vi "ATF-P&ID v2.vi"() -> ()   [LabVIEW 2022 SP3]
panel:
  in  "Exit":bool
  out "Boolean 73":bool
  out "Boolean 30":bool
  in  "F EPV 1008":bool
  out "NC EPV 1008 HSS":bool
  out "Boolean 27":bool
  in  "F EPV 1007":bool
  out "F EPV 1007 HSS":bool
  in  "F EPV 1004":bool
  out "NC EPV 1004 HSS":bool
  out "Boolean 26":bool
  in  "NC EPV 1001":bool
  out "NC EPV 1001 HSS":bool
  out "Boolean 23":bool
  out "Boolean 25":bool
  out "NO EPV 477 HSS  3":bool
  in  "NC EPV 61":bool
  out "Boolean 104":bool
  out "Boolean 47":bool
  out "Boolean 3":bool
  out "Boolean 24":bool
  out "NC EPV 56 HSS":bool
  in  "NC EPV 56":bool
  out "Boolean 16":bool
  out "Boolean 116":bool
  in  "NO EPV 122":bool
  out "Boolean 46":bool
  out "NO EPV 1102 HSS 2":bool
  out "Boolean 103":bool
  out "F_RTD_56(K)":dbl format="%.2g"
  out "N_PT_121":dbl format="%.2g"
  out "WTT_LS 2":dbl(slide) scale=0.1..100.0
  out "Boolean 71":bool
  out "F_RTD_1013 (K)":dbl format="%.2g"
  out "PT SC":dbl format="%.2g"
  out "W_RTD_1177 (K)":dbl format="%.2g"
  out "F_SC_RTD(K)":dbl format="%.2g"
  out "PT 1000(K)":dbl format="%.2g"
  out "PT 1000-2 (K)":dbl format="%.2g"
  out "F_PT_1013b (bar)":dbl format="%.2g"
  out "F_PT_1013a (bar)":dbl format="%.2g"
  out "F_PT_1019":dbl format="%.2g"
  out "F_TCV_1018":dbl format="%.2g"
  out "TCV_1018(FB) %":dbl format="%.2g"
  out "Boolean 108":bool
  out "Boolean 107":bool
  out "F_RTD_1011(K)":dbl format="%.2g"
  out "Boolean 21":bool
  out "Boolean 138":bool
  out "Boolean 29":bool
  out "Boolean 28":bool
  out "F_PT_1011a (bar)":dbl format="%.2g"
  out "F_PT_1011b (bar)":dbl format="%.2g"
  out "F_FM_1010 (kg/s)":dbl format="%.2g"
  out "Boolean 106":bool
  out "Boolean 105":bool
  out "Boolean 121":bool
  out "Boolean 126":bool
  out "Boolean 109":bool
  out "Boolean 6":bool
  out "Boolean 81":bool
  out "NO EPV 477 HSS  2":bool
  in  "NO EPV 477":bool
  in  "NO EPV 478R":bool
  out "NO EPV 1207 HSS 2":bool
  out "Boolean 54":bool
  out "Boolean 53":bool
  out "Boolean 22":bool
  out "Boolean 86":bool
  out "F_PT_56 _R":dbl format="%.2g"
  in  "NC EPV 481":bool
  out "NC EPV 481 HSS":bool
  out "Boolean 85":bool
  out "F_PT_56":dbl format="%.2g"
  out "Boolean 115":bool
  out "Boolean 52":bool
  out "N_PT_480":dbl format="%.2g"
  out "Boolean 120":bool
  out "Boolean 72":bool
  out "Boolean 119":bool
  out "Boolean 13":bool
  out "N_PT_ATF_Cyl":dbl format="%.2g"
  out "Boolean 83":bool
  out "Boolean 102":bool
  out "Boolean 82":bool
  out "Boolean 101":bool
  out "N_PT_1101":dbl format="%.2g"
  out "N_PT_1090   2":dbl format="%.2g"
  in  "N EPV 1091":bool
  out "NO EPV 1091 HSS":bool
  out "Boolean 20":bool
  out "Boolean 118":bool
  in  "NC EPV 1217":bool
  out "NC EPV 1217 HSS":bool
  out "Boolean 4":bool
  out "Boolean 114":bool
  out "Boolean 12":bool
  out "N_PT_Water_Cyl":dbl format="%.2g"
  out "Boolean 79":bool
  out "N_PT_1210":dbl format="%.2g"
  out "Boolean 117":bool
  out "W_PT_1212":dbl format="%.2g"
  out "W_RTD_1212(K)":dbl format="%.2g"
  out "Boolean 19":bool
  out "Boolean 18":bool
  out "Boolean 8":bool
  out "Boolean 15":bool
  out "Boolean 14":bool
  out "Boolean 11":bool
  out "Boolean 10":bool
  in  "NO EPV 1207":bool
  out "Boolean 7":bool
  out "Boolean 5":bool
  in  "NC EPV 1214":bool
  out "Boolean 141":bool
  out "Boolean 9":bool
  out "WTT_LS":dbl(slide) scale=0.1..100.0
  out "Boolean 140":bool
  out "Boolean 144":bool
  out "Boolean 128":bool
  out "Boolean 125":bool
  in  "NO EPV 1102":bool
  out "Boolean 45":bool
  out "NC EPV 1211 HSS":bool
  in  "NC EPV 1211":bool
  out "NO EPV 1207 HSS":bool
  out "NC EPV 1214 HSS":bool
  out "NO EPV 1102 HSS":bool
  out "Boolean 113":bool
  out "Boolean 2":bool
  out "Boolean 100":bool
  out "Boolean 80":bool
  out "Boolean 78":bool
  out "Boolean 70":bool
  out "Boolean":bool
  out "Boolean 51":bool
  out "Boolean 17":bool
  out "Boolean 112":bool
  out "Sampling Rate_Accelerometer":dbl
  # "ATF PUMP & STORAGE P&ID"
  # "WTT\nh(mm)"
  # "ATF"
  # "ATF"
  # "ATF STORAGE\nAREA"
  # "ATF PUMP\nAREA"
  # "GN2"
  # "GN2"
  # "Version:V0.1"
  # "Release Date:14/10/2024"
  # "GN2"
  # "GN2"
  # "GN2"
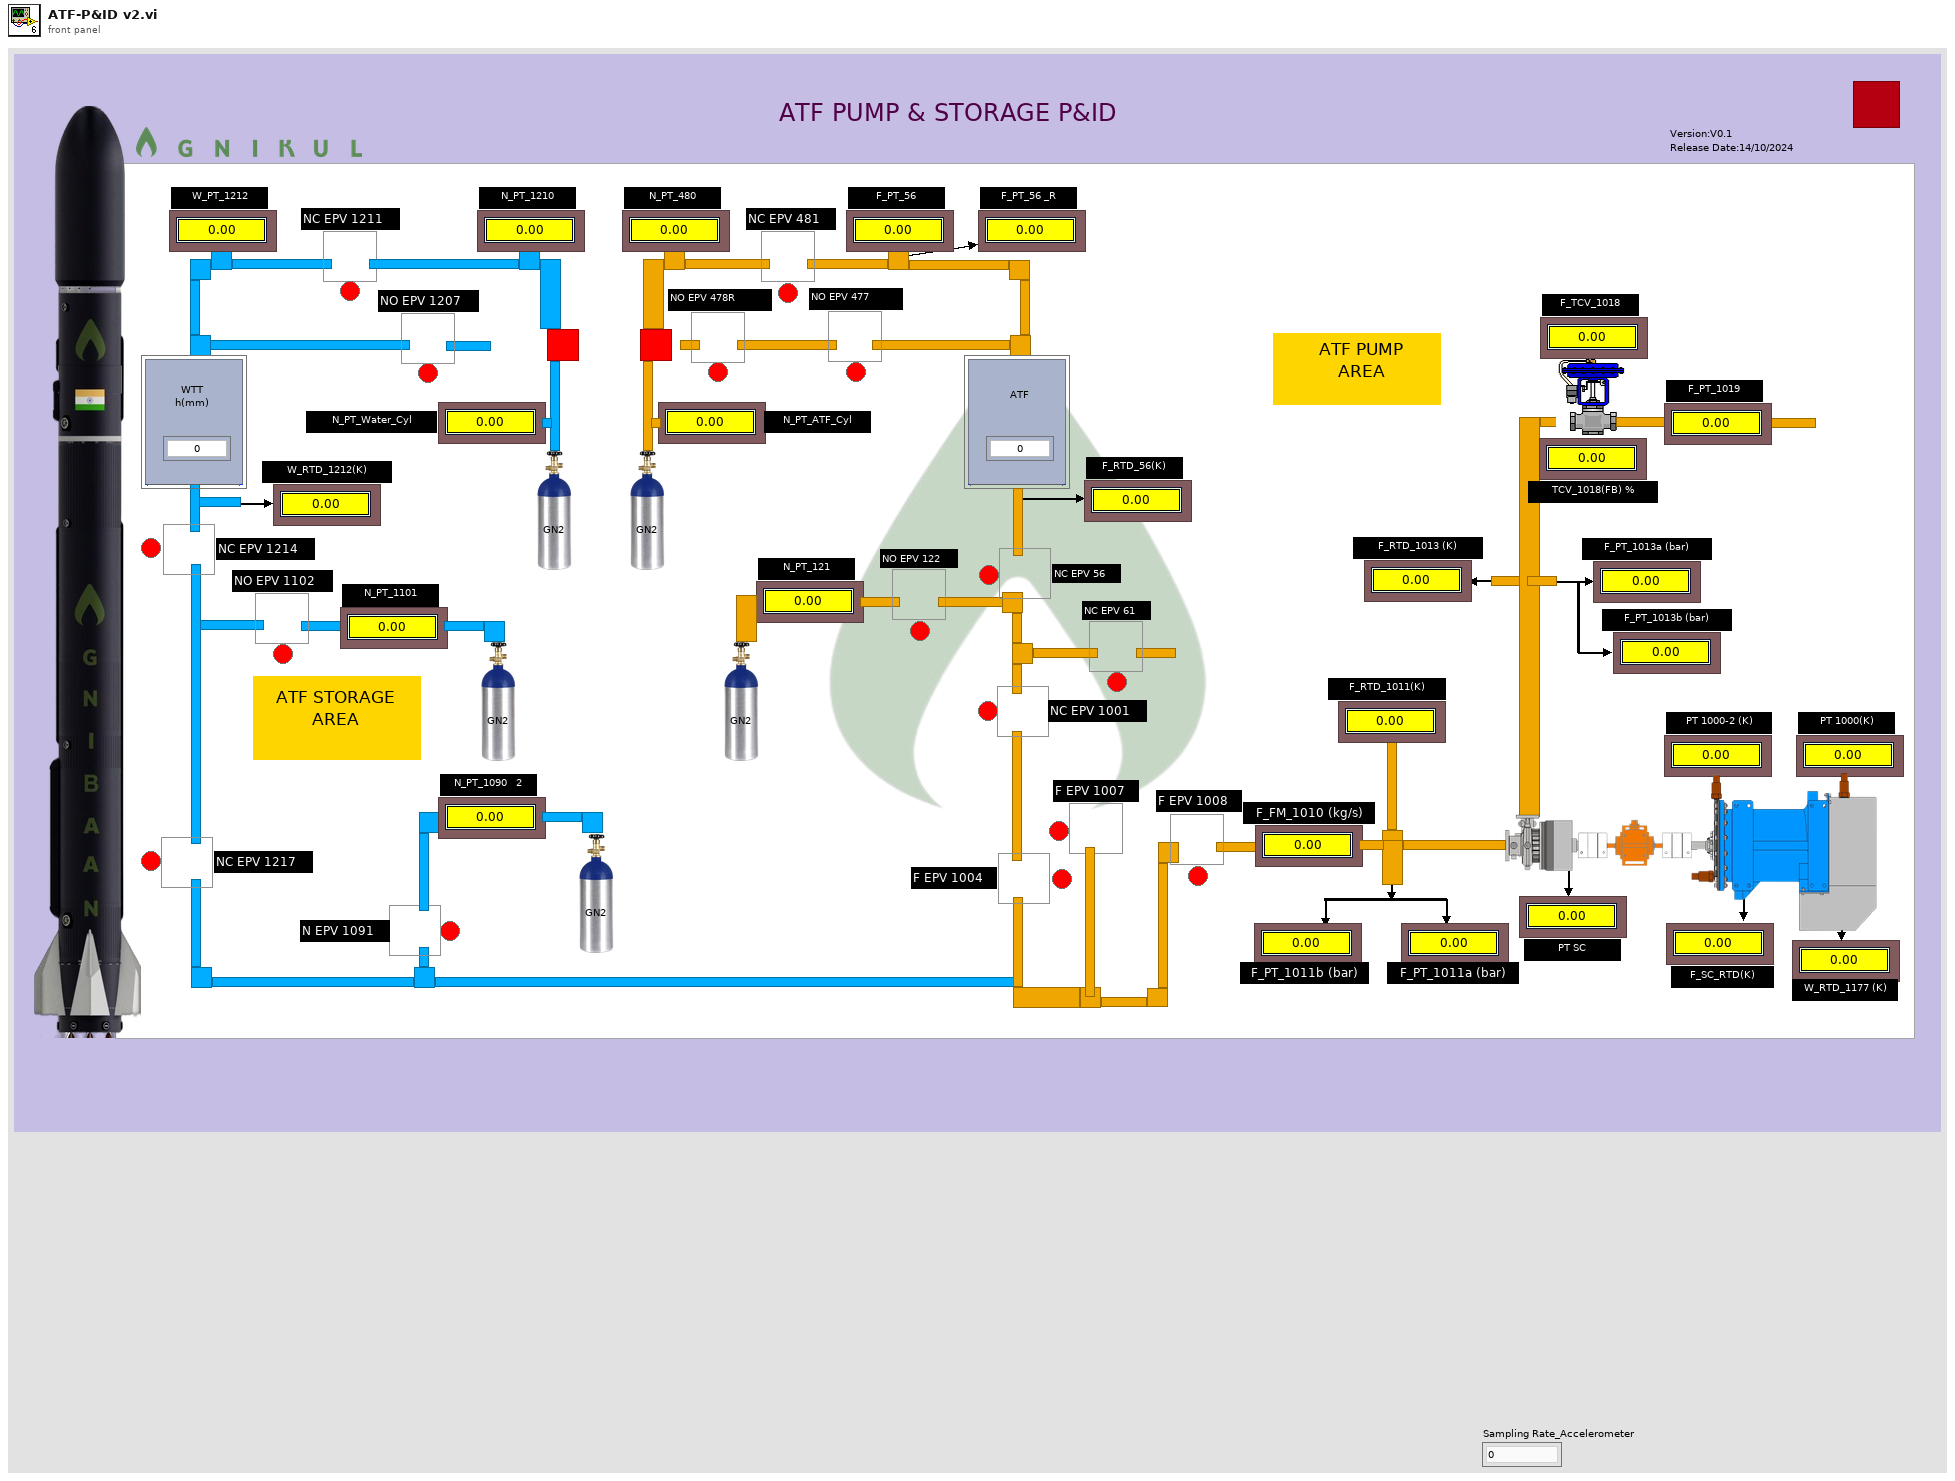
[diagram p1: front panel]
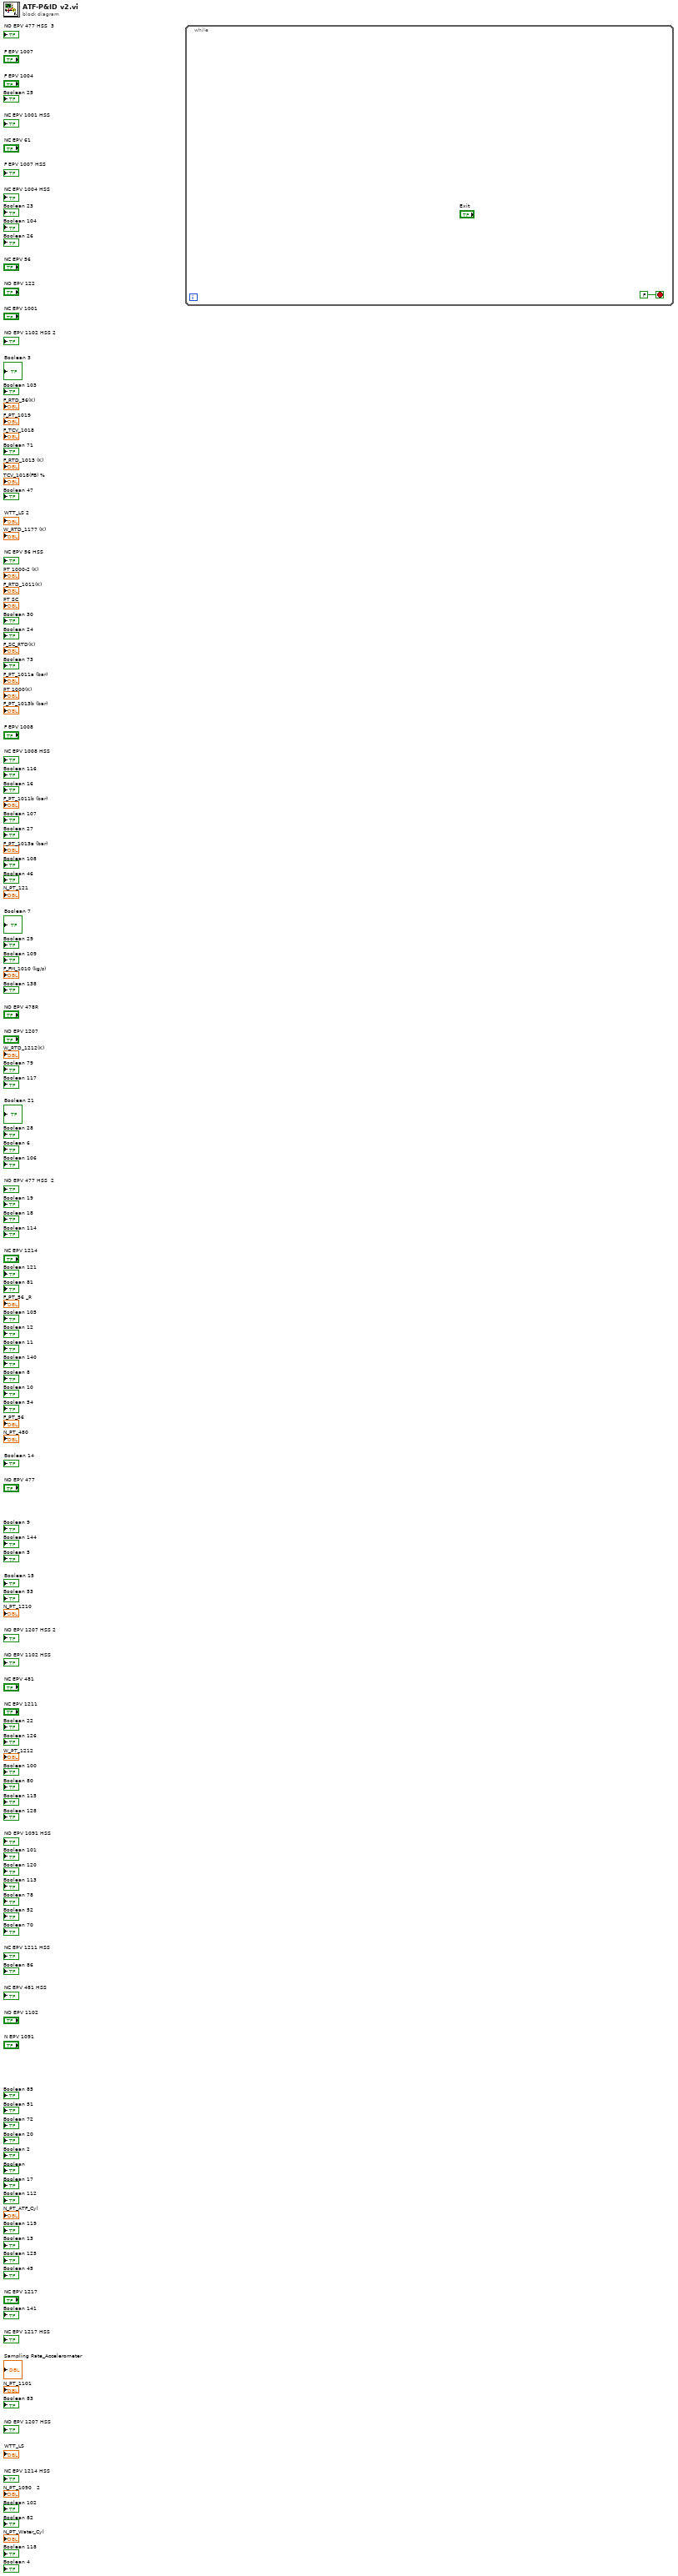
[diagram p0: block diagram]
diagram:
  n1 = while {
    stop <- FALSE stop-if-true
  }
